vi "7_11_Fxp_addation.vi"(1 "y":fxp<+/-,11,7>, 2 "x":fxp<+/-,11,7>) -> (0 "x+y":fxp<+/-,12,8> format="%.41g")   [LabVIEW 2020]
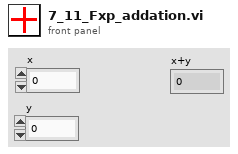
[diagram p1: front panel]
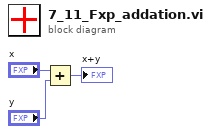
[diagram p0: block diagram]
diagram:
  n1 = Add(x="x", y="y") -> (x+y=→"x+y":fxp<+/-,12,8>)
